vi "Close Ports A.vi"(11 "GIC Input":T1={"     Use ?\nOff       On"=[FALSE, TRUE, FALSE, TRUE], "Mode:"=FALSE, "WP Data"="", "Hokuyo Port"="COM7", "Prop  Port"="COM6", "Compass Port"="", "GPS Port"="", "Num of WPs"=0, "WP Lats and Longs"={"WP Lats"=[], "WP Longs"=[]}, "Obst Lats and Longs"={"Obst Lats"=[], "Obst Longs"=[]}, "Parameters"=[], "GPS Data"=[], "Compass"=0.0, "LMS Vector"=[], "Vision Vector"=[], "Direction Cmd"=0.0, "Speed Cmd"=0.0, "WP Vector"=[], "WP Number"=0, "Extra"=0, "SW Map"=[], "Path Cluster"={"Path x node"=[], "Path y node"=[]}} {"Obst Lats and Longs"."Obst Longs" format="%#_8g"; "Obst Lats and Longs"."Obst Lats" format="%#_8g"}) -> ()   [LabVIEW 2014]
uses:
  Hokuyo URG Series.lvlib
panel:
  # "Close Ports A"
  # "Input:"
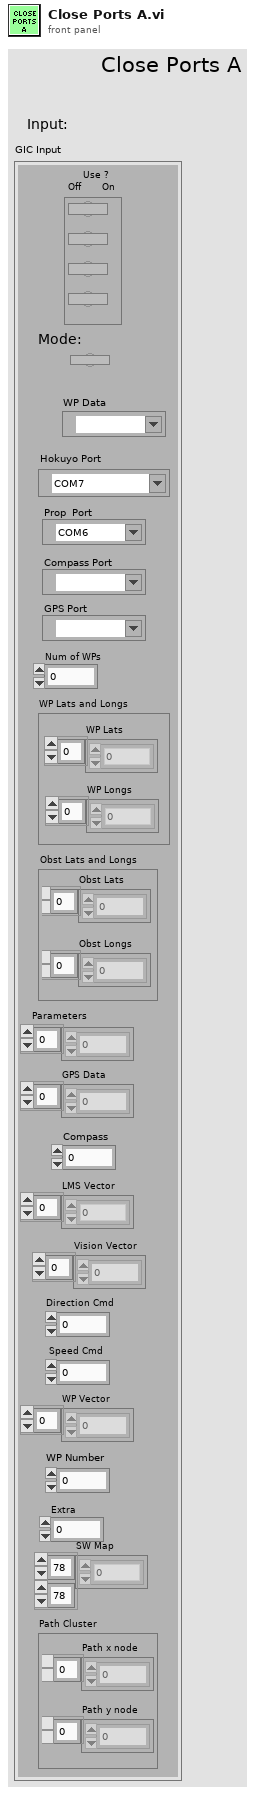
[diagram p1: front panel]
types:
  T1 = cluster{"     Use ?\nOff       On":bool[], "Mode:":bool, "WP Data":refnum<visa-resource-name>, "Hokuyo Port":refnum<visa-resource-name>, "Prop  Port":refnum<visa-resource-name>, "Compass Port":refnum<visa-resource-name>, "GPS Port":refnum<visa-resource-name>, "Num of WPs":i16, "WP Lats and Longs":cluster{"WP Lats":dbl[], "WP Longs":dbl[]}, "Obst Lats and Longs":cluster{"Obst Lats":dbl[], "Obst Longs":dbl[]}, "Parameters":dbl[], "GPS Data":dbl[], "Compass":dbl, "LMS Vector":dbl[], "Vision Vector":dbl[], "Direction Cmd":dbl, "Speed Cmd":dbl, "WP Vector":dbl[], "WP Number":i32, "Extra":i16, "SW Map":i32[][], "Path Cluster":cluster{"Path x node":dbl[], "Path y node":dbl[]}}
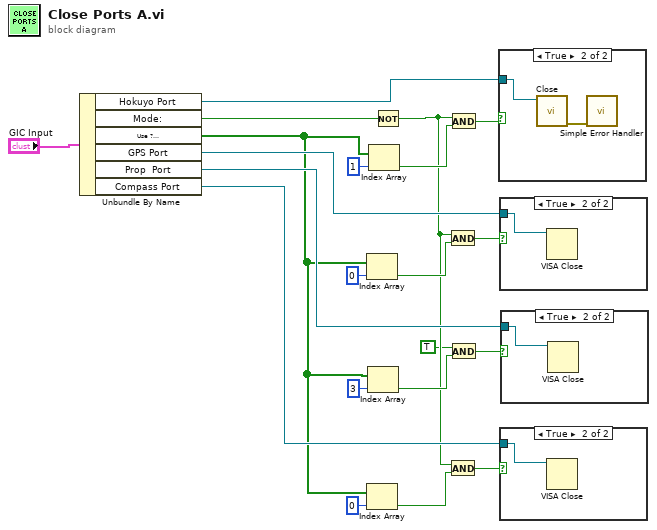
[diagram p0: block diagram]
diagram:
  n1 = Unbundle By Name("GIC Input") -> ("Hokuyo Port"=w18:refnum<visa-resource-name>, "Mode:"=w16:bool, "Use ?\nOff       On"=w3:bool[], "GPS Port"=w12:refnum<visa-resource-name>, "Prop  Port"=w8:refnum<visa-resource-name>, "Compass Port"=w4:refnum<visa-resource-name>)
  n2 = Index Array(array=w3, index=0) -> (element=w13:bool)
  n3 = Index Array(array=w3, index=0) -> (element=w5:bool)
  n4 = Index Array(array=w3, index=3) -> (element=w9:bool)
  n5 = Index Array(array=w3, index=1) -> (element=w20:bool)
  n6 = Not(x=w16) -> (.not. x?=w2:bool)
  n7 = And(x=w2, y=w13) -> (x .and. y?=w14:bool)
  n8 = And(x=w2, y=w5) -> (x .and. y?=w6:bool)
  n9 = And(x=w2, y=w20) -> (x .and. y?=w19:bool)
  n10 = And(x=TRUE, y=w9) -> (x .and. y?=w10:bool)
  n11 = case shown="True" w19 {
    tunnel: w18 -> [_ w22]
    frame False {
    }
    frame True {
      n12 = call "Close.vi"("VISA resource name"=w22) -> ("error out"=w23:errorcluster)  [unwired: 10 in]
      n13 = call <vilib>:"Simple Error Handler.vi"("error in (no error)"=w23) -> ()  [unwired: 4 in, 5 out]
    }
  }
  n14 = case shown="True" w14 {
    tunnel: w12 -> [_ w24]
    frame False {
    }
    frame True {
      n15 = VISA Close(VISA resource name=w24) -> ()  [unwired: 1 in, 1 out]
    }
  }
  n16 = case shown="True" w6 {
    tunnel: w4 -> [_ w25]
    frame False {
    }
    frame True {
      n17 = VISA Close(VISA resource name=w25) -> ()  [unwired: 1 in, 1 out]
    }
  }
  n18 = case shown="True" w10 {
    tunnel: w8 -> [_ w26]
    frame False {
    }
    frame True {
      n19 = VISA Close(VISA resource name=w26) -> ()  [unwired: 1 in, 1 out]
    }
  }
